vi "Read E5071C_VISA.vi"(8 "error in (no error)":errorcluster, 11 "E5071C in":refnum<class "E5071C.lvclass">) -> (0 "error out":errorcluster, 2 "E5071C_VISA":refnum<visa-resource-name>, 3 "E5071C out":refnum<class "E5071C.lvclass">)   [LabVIEW 2020, in "E5071C.lvlib" / "E5071C.lvclass"]
uses:
  E5071C.lvclass
  E5071C.lvclass/E5071C.ctl
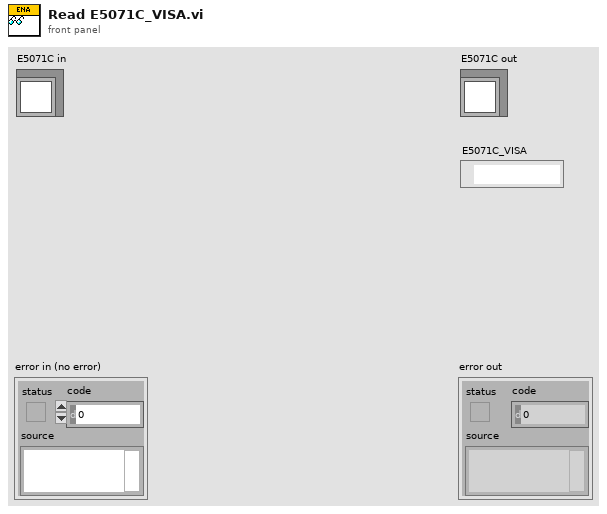
[diagram p1: front panel]
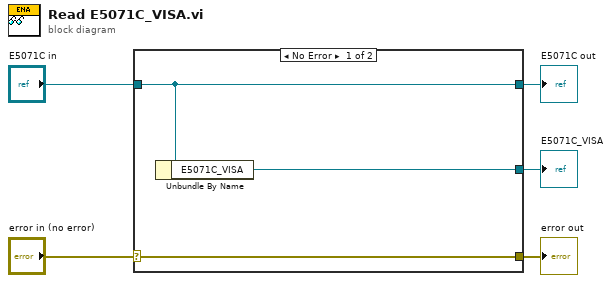
[diagram p0: block diagram]
diagram:
  n1 = case shown="No Error" "error in (no error)" {
    selector: "error in (no error)" -> [w8 w9]
    tunnel: [w8 w9] -> w4
    tunnel: [w7 w10] -> w2
    tunnel: "E5071C in" -> [w7 w10]
    tunnel: [w6 _] -> w1
    frame No Error {
      n2 = Unbundle By Name(w7) -> ("E5071C_VISA"=w6:refnum<visa-resource-name>)
    }
    frame Error {
    }
  }
  "error out" <- w4
  "E5071C out" <- w2
  "E5071C_VISA" <- w1
